vi "Sea-Level SWI Array of States to Ports.vi"(2 "State Array":bool[](array[boolean]), 3 "Number of Ports":i8=4) -> (0 "SWI Position":T1)   [LabVIEW 2011]
uses:
  TypeDefs/Sea-Level SWI Position.ctl
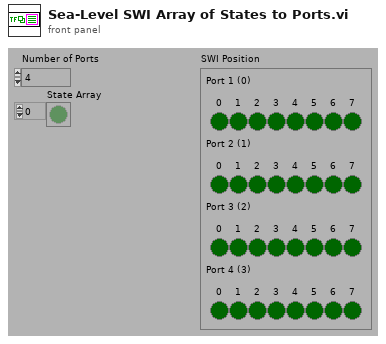
[diagram p1: front panel]
types:
  T1 = typedef "Sea-Level SWI Position.ctl" = cluster{"Port 1 (0)":cluster{"0":bool, "1":bool, "2":bool, "3":bool, "4":bool, "5":bool, "6":bool, "7":bool}, "Port 2 (1)":cluster{"0":bool, "1":bool, "2":bool, "3":bool, "4":bool, "5":bool, "6":bool, "7":bool}, "Port 3 (2)":cluster{"0":bool, "1":bool, "2":bool, "3":bool, "4":bool, "5":bool, "6":bool, "7":bool}, "Port 4 (3)":cluster{"0":bool, "1":bool, "2":bool, "3":bool, "4":bool, "5":bool, "6":bool, "7":bool}}
  T2 = cluster{"[0]":bool, "[1]":bool, "[2]":bool, "[3]":bool, "[4]":bool, "[5]":bool, "[6]":bool, "[7]":bool}
  T3 = cluster{"[0]":cluster{"[0]":bool, "[1]":bool, "[2]":bool, "[3]":bool, "[4]":bool, "[5]":bool, "[6]":bool, "[7]":bool}, "[1]":cluster{"[0]":bool, "[1]":bool, "[2]":bool, "[3]":bool, "[4]":bool, "[5]":bool, "[6]":bool, "[7]":bool}, "[2]":cluster{"[0]":bool, "[1]":bool, "[2]":bool, "[3]":bool, "[4]":bool, "[5]":bool, "[6]":bool, "[7]":bool}, "[3]":cluster{"[0]":bool, "[1]":bool, "[2]":bool, "[3]":bool, "[4]":bool, "[5]":bool, "[6]":bool, "[7]":bool}}
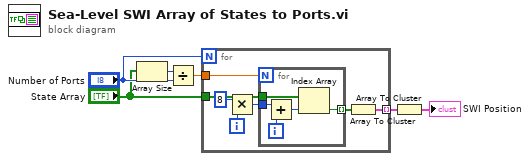
[diagram p0: block diagram]
diagram:
  n1 = Array Size(array="State Array") -> (size(s)=w6:i32)
  n2 = Divide(x=w6, y="Number of Ports") -> (x/y=w3:dbl)
  n3 = for {
    N: "Number of Ports" -> [_]
    tunnel: "State Array" -> [w13]
    tunnel: w3 -> [w12]
    tunnel: [w7] -> w2 mode=indexing
    i -> [w10]
    n4 = Multiply(x=8, y=w10) -> (x*y=w11:i32)
    n5 = for {
      N: w12 -> [_]
      tunnel: w13 -> [w18]
      tunnel: w11 -> [w16]
      tunnel: [w14] -> w8 mode=indexing
      i -> [w17]
      n6 = Add(x=w16, y=w17) -> (x+y=w15:i32)
      n7 = Index Array(array=w18, index=w15) -> (element=w14:bool)
    }
    n8 = Array To Cluster(array=w8) -> (cluster=w7:T2)
  }
  n9 = Array To Cluster(array=w2) -> (cluster=→"SWI Position":T3)
